vi "Gyro.vi"() -> ()   [LabVIEW 2019]
uses:
  <vilib>/MakerHub/LINX/Public/Sensors/Accelerometer/MPU60X0/DeviceAddresses.ctl
  <vilib>/MakerHub/LINX/Public/Utilities/Open Serial.vi
  <vilib>/picture/3D Picture Control/Object/Create Object (name).vi
  <vilib>/MakerHub/LINX/LMH-LINX.lvlib
  <vilib>/MakerHub/LINX/Public/Sensors/Accelerometer/MPU60X0/MPU60X0.lvlib
  <vilib>/picture/3D Picture Control/NI_3D Picture Control.lvlib
  <vilib>/Analysis/NI_AALPro.lvlib
panel:
  out "3D Picture":refnum<vi>(3d-picture)
  in  "?":bool
  out "Gyro  Data (dps)":T1
  out "Acceleration Data (g)":T1
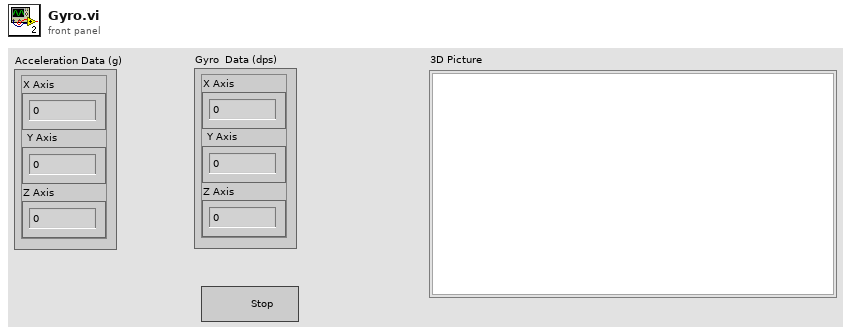
[diagram p1: front panel]
types:
  T1 = cluster{"X Axis":i16, "Y Axis":i16, "Z Axis":i16}
  T2 = typedef "LMH-LINX.lvlib/MPU60X0.lvlib/DeviceAddresses.ctl" = enum16{"0x68", "0x69"}
  T3 = typedef "LMH-LINX.lvlib/LINX Ref.ctl" = cluster{"IO":T4, "Interface":T5, "LINX Device Config":T6}
  T4 = typedef "LMH-LINX.lvlib/Platform.ctl" = enum16{"Remote", "Local"}
  T5 = typedef "LMH-LINX.lvlib/Interface.ctl" = enum16{"Serial", "TCP"}
  T6 = typedef "LMH-LINX.lvlib/Device.lvlib/LINX Device Config.ctl" = cluster{"Interface":T5, "COM Port":refnum<visa-resource-name>, "TCP Configuration":T7, "Device Family":u8, "Device ID":u8, "Device Name":string, "TCP Ref":refnum<k5>, "Channels":T8}
  T7 = typedef "LMH-LINX.lvlib/Device.lvlib/TCP Config.ctl" = cluster{"IP Address":string, "Port":u16}
  T8 = typedef "LMH-LINX.lvlib/Channels.ctl" = cluster{"DI":u8[], "DO":u8[], "AI":u8[], "AO":u8[], "PWM":u8[], "QE":u8[], "UART":u8[], "I2C 2":u8[], "SPI":u8[], "CAN":u8[], "Servo":u8[], "AI Ref (V)":dbl, "AI Resolution (Bits)":u8, "AO Ref (V)":dbl, "AO Resolution (Bits)":u8}
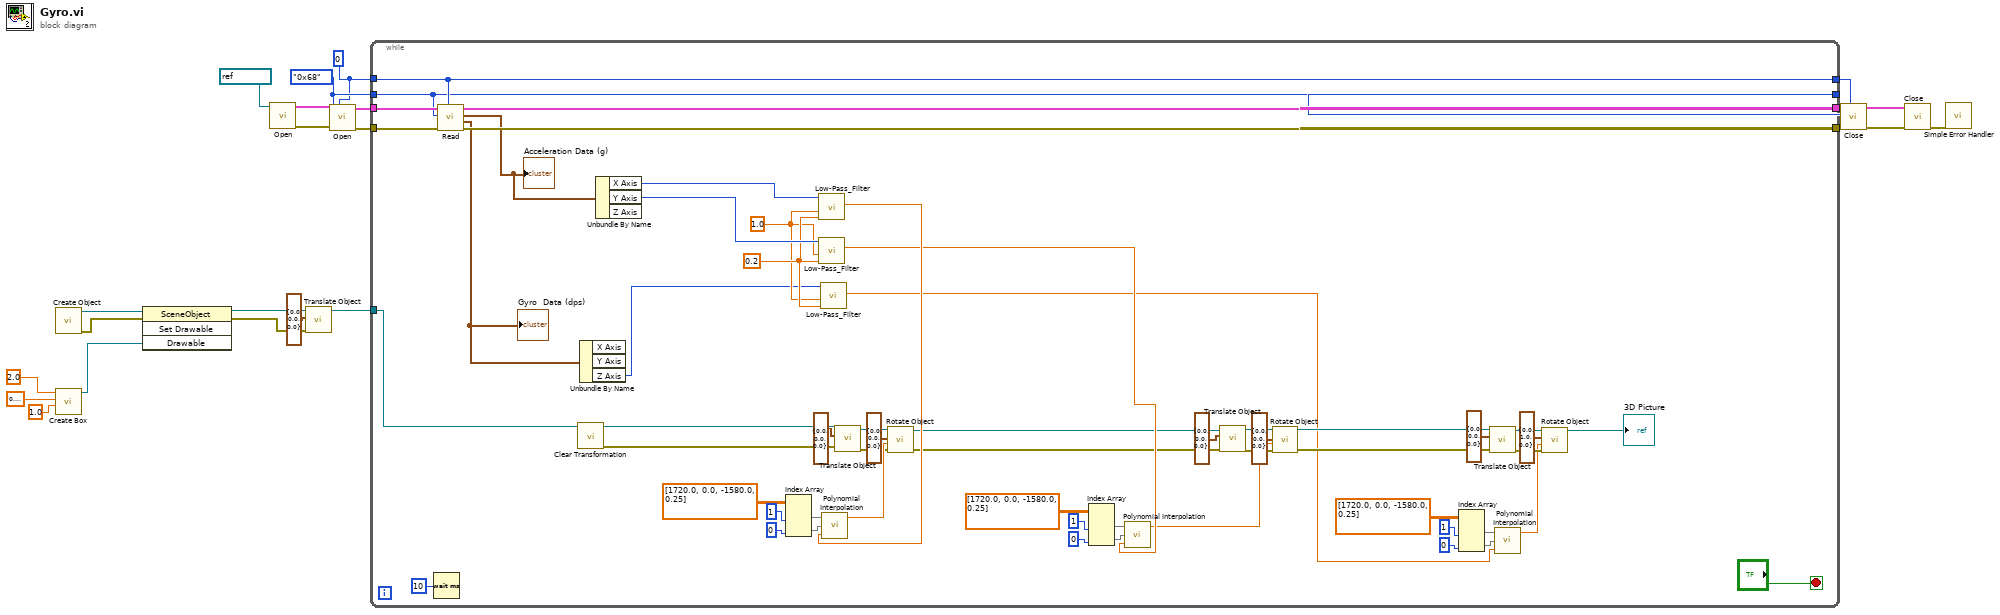
[diagram p0: block diagram]
diagram:
  w5 = u8 0 ("I2C Channel")
  w15 = DeviceAddresses."0x68" ("I2C Slave Address")
  n1 = call-poly <vilib>:"Create Object.vi"() -> ("error out"=w8:errorcluster, "Scene:New Object"=w11:refnum<vi>)  [unwired: 10 in]
  n2 = call <vilib>:"Create Box.vi"("Length Z"=sgl 1.0, "Length Y"=sgl 0.2, "Length X"=sgl 2.0) -> ("New Box Refnum"=w7:refnum<vi>)  [unwired: 7 in, 1 out]
  n3 = invoke class="SceneObject" method="Set Drawable"(reference=w11, error in=w8, "Drawable"=w7) -> (reference out=w10:refnum<vi>, error out=w9:errorcluster)  [unwired: 1 in, 2 out]
  n4 = call-poly <vilib>:"Open.vi"("Serial Port"=refnum<visa-resource-name> "COM9") -> ("Error Out"=w23:errorcluster, "LINX Resource"=w24:T3)  [unwired: 8 in, 1 out]
  n5 = call <vilib>:"Translate Object.vi"("error in (no error)"=w9, "Translation"=cluster{"X":sgl, "Y":sgl, "Z":sgl} {"X"=0.0, "Y"=0.0, "Z"=0.0}, "Scene.Object In"=w10) -> ("Scene.Object Out"=w3:refnum<vi>)  [unwired: 7 in, 1 out]
  n6 = call <vilib>:"Open.vi"("I2C Channel"=w5, "Error In"=w23, "I2C Slave Address"=w15, "LINX Resource"=w24) -> ("Error Out"=w20:errorcluster, "LINX Resource"=w21:T3)  [unwired: 6 in]
  n7 = while {
    tunnel: w21 -> [w80]
    tunnel: w20 -> [w79]
    tunnel: [w78] -> w18
    tunnel: [w77] -> w19
    tunnel: w15 -> [w72]
    tunnel: w5 -> [w73]
    tunnel: [w73] -> w4
    tunnel: [w72] -> w1
    tunnel: w3 -> [w69]
    stop <- "?" stop-if-true
    w60 = 0.2 ("Ts")
    w59 = 1.0 ("Tf")
    n8 = Wait (ms)(milliseconds to wait=u32 10) -> ()  [unwired: 1 out]
    n9 = call <vilib>:"Read.vi"("I2C Channel"=w73, "Error In"=w79, "I2C Slave Address"=w72, "LINX Resource"=w80) -> ("Error Out"=w77:errorcluster, "Gyro  Data (dps)"=w57:T1, "Acceleration Data (g)"=w75:T1, "LINX Resource"=w78:T3)  [unwired: 3 in, 1 out]
    "Acceleration Data (g)" <- w75
    "Gyro  Data (dps)" <- w57
    n10 = call <vilib>:"Clear Transformation.vi"("Object Refnum In"=w69) -> ("error out"=w44:errorcluster, "Object Refnum Out"=w43:refnum<vi>)  [unwired: 9 in]
    n11 = Unbundle By Name(w57) -> ("Z Axis"=w56:i16)  [unwired: 2 out]
    n12 = Unbundle By Name(w75) -> ("X Axis"=w68:i16, "Y Axis"=w67:i16)  [unwired: 1 out]
    n13 = Index Array(array=dbl[][] [[1720.0, 0.0], [-1580.0, 0.25]], index (col) #1=1 ("disabled index (col)"), index (col) #2=0 ("index (col)")) -> (element #1=w51:dbl[], element #2=w52:dbl[])  [unwired: 2 in]
    n14 = call "Low-Pass_Filter.vi"("Ts"=w60, "Tf"=w59, "Input"=w68) -> ("Filter Output"=w71:dbl)  [unwired: 6 in]
    n15 = call "Low-Pass_Filter.vi"("Ts"=w60, "Tf"=w59, "Input"=w67) -> ("Filter Output"=w70:dbl)  [unwired: 6 in]
    n16 = call "Low-Pass_Filter.vi"("Ts"=w60, "Tf"=w59, "Input"=w56) -> ("Filter Output"=w26:dbl)  [unwired: 6 in]
    n17 = call <vilib>:"Polynomial Interpolation.vi"("x value"=w71, "X"=w52, "Y"=w51) -> ("interpolation value"=w55:dbl)  [unwired: 2 out]
    n18 = call <vilib>:"Translate Object.vi"("error in (no error)"=w44, "Translation"=cluster{"X":sgl, "Y":sgl, "Z":sgl} {"X"=0.0, "Y"=0.0, "Z"=0.0}, "Scene.Object In"=w43) -> ("error out"=w46:errorcluster, "Scene.Object Out"=w45:refnum<vi>)  [unwired: 7 in]
    n19 = call <vilib>:"Rotate Object.vi"("error in (no error)"=w46, "Angle"=w55, "Axis"=cluster{"X":sgl, "Y":sgl, "Z":sgl} {"X"=0.0, "Y"=0.0, "Z"=0.0}, "Scene.Object In"=w45) -> ("error out"=w50:errorcluster, "Scene.Object Out"=w47:refnum<vi>)  [unwired: 6 in]
    n20 = Index Array(array=dbl[][] [[1720.0, 0.0], [-1580.0, 0.25]], index (col) #1=1 ("disabled index (col)"), index (col) #2=0 ("index (col)")) -> (element #1=w53:dbl[], element #2=w54:dbl[])  [unwired: 2 in]
    n21 = call <vilib>:"Polynomial Interpolation.vi"("x value"=w70, "X"=w54, "Y"=w53) -> ("interpolation value"=w32:dbl)  [unwired: 2 out]
    n22 = call <vilib>:"Translate Object.vi"("error in (no error)"=w50, "Translation"=cluster{"X":sgl, "Y":sgl, "Z":sgl} {"X"=0.0, "Y"=0.0, "Z"=0.0}, "Scene.Object In"=w47) -> ("error out"=w49:errorcluster, "Scene.Object Out"=w48:refnum<vi>)  [unwired: 7 in]
    n23 = call <vilib>:"Rotate Object.vi"("error in (no error)"=w49, "Angle"=w32, "Axis"=cluster{"X":sgl, "Y":sgl, "Z":sgl} {"X"=0.0, "Y"=0.0, "Z"=0.0}, "Scene.Object In"=w48) -> ("error out"=w63:errorcluster, "Scene.Object Out"=w64:refnum<vi>)  [unwired: 6 in]
    n24 = Index Array(array=dbl[][] [[1720.0, 0.0], [-1580.0, 0.25]], index (col) #1=1 ("disabled index (col)"), index (col) #2=0 ("index (col)")) -> (element #1=w30:dbl[], element #2=w31:dbl[])  [unwired: 2 in]
    n25 = call <vilib>:"Translate Object.vi"("error in (no error)"=w63, "Translation"=cluster{"X":sgl, "Y":sgl, "Z":sgl} {"X"=0.0, "Y"=0.0, "Z"=0.0}, "Scene.Object In"=w64) -> ("error out"=w65:errorcluster, "Scene.Object Out"=w66:refnum<vi>)  [unwired: 7 in]
    n26 = call <vilib>:"Polynomial Interpolation.vi"("x value"=w26, "X"=w31, "Y"=w30) -> ("interpolation value"=w25:dbl)  [unwired: 2 out]
    n27 = call <vilib>:"Rotate Object.vi"("error in (no error)"=w65, "Angle"=w25, "Axis"=cluster{"X":sgl, "Y":sgl, "Z":sgl} {"X"=0.0, "Y"=1.0, "Z"=0.0}, "Scene.Object In"=w66) -> ("Scene.Object Out"=→"3D Picture":refnum<vi>)  [unwired: 6 in, 1 out]
  }
  n28 = call <vilib>:"Close.vi"("I2C Channel (0)"=w4, "Error In"=w19, "I2C Slave Address (0)"=w1, "LINX Resource"=w18) -> ("Error Out"=w16:errorcluster, "LINX Resource"=w17:T3)  [unwired: 6 in]
  n29 = call <vilib>:"Close.vi"("Error In"=w16, "LINX Resource"=w17) -> ("Error Out"=w2:errorcluster)  [unwired: 9 in]
  n30 = call <vilib>:"Simple Error Handler.vi"("error in (no error)"=w2) -> ()  [unwired: 4 in, 5 out]
